vi "DECIMATION_PATTERN - Type.vi"(8 "error in (no error)":errorcluster) -> (0 "error out":errorcluster, 3 "DECIMATION_PATTERN_VALUE":i32)   [LabVIEW 2013]
doc: "<b>Buffer policy settings can be only unsafe in xiAPI LabVIEW library</b>\nUNSAFE : User gets pointer to internally allocated circle buffer and data may be overwritten by device.\nSAFE : Data from device will be copied to user allocated buffer or xiApi allocated memory."
uses:
  DECIMATION_PATTERN.ctl
  C:/Projects/Cameras3.x/xiLib/xiLIB_64bit/xiLIB/xiCamLib/API/x64/xiApi.NETX64.dll
  xiLIB_64bit/xiLIB/xiCamLib/API/x64/xiApi.NETX64.dll
panel:
  in  "DECIMATION_PATTERN":T1
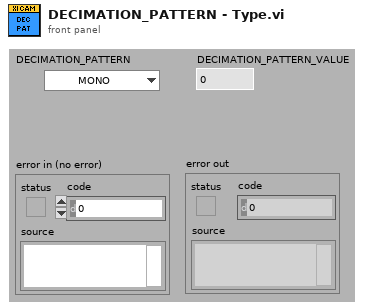
[diagram p1: front panel]
types:
  T1 = typedef "DECIMATION_PATTERN.ctl" = enum16{"MONO", "BAYER"}
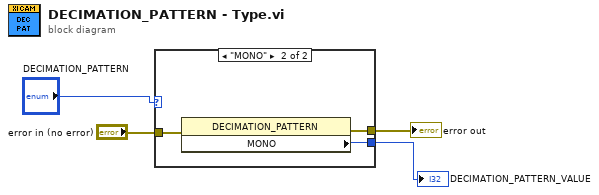
[diagram p0: block diagram]
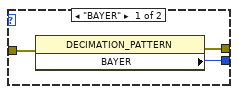
[diagram p2: hidden frame]
diagram:
  n1 = case shown="\"MONO\"" "DECIMATION_PATTERN" {
    tunnel: "error in (no error)" -> [w7 w10]
    tunnel: [w6 w9] -> w3
    tunnel: [w5 w8] -> w2
    frame "BAYER" {
      n2 = property class="DECIMATION_PATTERN"(error in=w7) -> (error out=w6:errorcluster, "BAYER"=w5:i32)  [unwired: 1 in, 1 out]
    }
    frame "MONO" {
      n3 = property class="DECIMATION_PATTERN"(error in=w10) -> (error out=w9:errorcluster, "MONO"=w8:i32)  [unwired: 1 in, 1 out]
    }
  }
  "error out" <- w3
  "DECIMATION_PATTERN_VALUE" <- w2
